vi "GetSibling_SequentialRead.vi"(8 "error in (no error)":errorcluster, 11 "node in":refnum<k20>) -> (0 "error out":errorcluster, 2 "node text":string, 3 "sibling node":refnum<k20>, 5 "node out":refnum<k20>)   [LabVIEW 2010, in "Pansino_XML_Read.lvlib"]
uses:
  Pansino_XML_Read.lvlib
  <vilib>/xml/NI_XML.lvlib
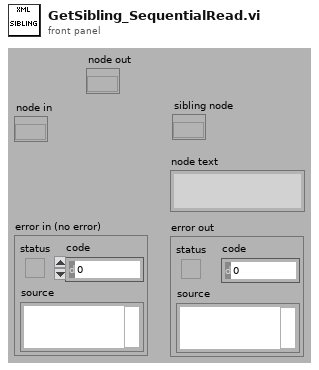
[diagram p1: front panel]
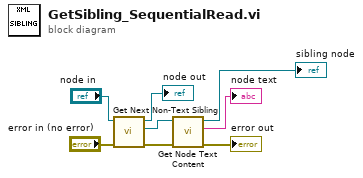
[diagram p0: block diagram]
diagram:
  n1 = call <vilib>:"Get Next Non-Text Sibling.vi"("error in (no error)"="error in (no error)", "node in"="node in") -> ("error out"=w8:errorcluster, "sibling node"=w7:refnum<k20>, "node out"=→"node out":refnum<k20>)  [unwired: 7 out]
  n2 = call <vilib>:"Get Node Text Content.vi"("error in (no error)"=w8, "node in"=w7) -> ("error out"=→"error out":errorcluster, "node text"=→"node text":string, "node out"=→"sibling node":refnum<k20>)  [unwired: 7 out]
